vi "while.vi"() -> ()   [LabVIEW 2020]
panel:
  out "Array":dbl[](array[numeric])
  out "Thermometer":dbl(slide) scale=0.0..100.0
  out "Numeric":i32
  in  "stop":bool
  # "While"
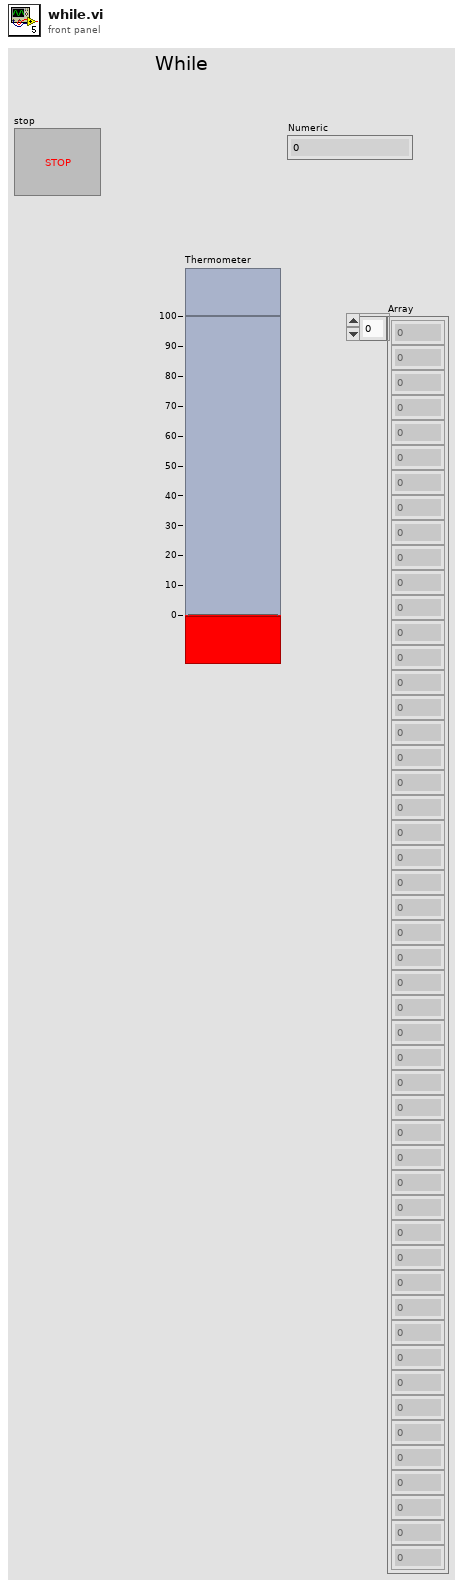
[diagram p1: front panel]
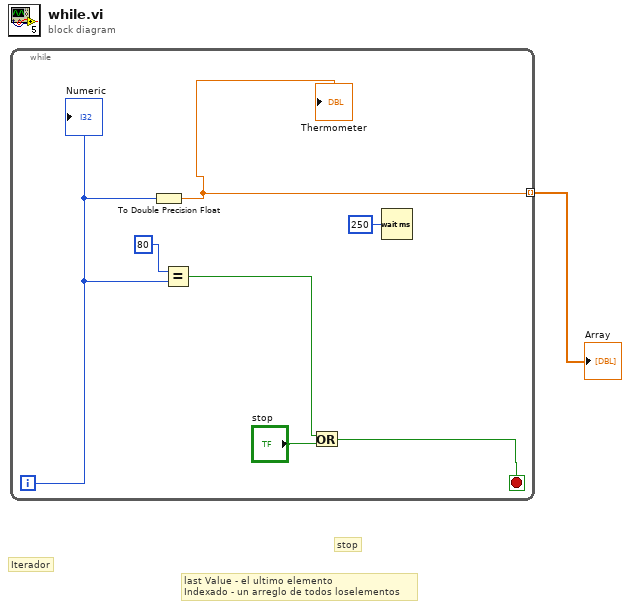
[diagram p0: block diagram]
diagram:
  # "last Value - el ultimo elemento\nIndexado - un arreglo de todos loselementos"
  # "stop"
  # "Iterador"
  n1 = while {
    tunnel: [w2] -> w1 mode=indexing
    i -> [w6]
    stop <- w3 stop-if-true
    n2 = To Double Precision Float(number=w6) -> (double precision float=w2:dbl)
    "Thermometer" <- w2
    n3 = Equal?(x=80, y=w6) -> (x = y?=w4:bool)
    n4 = Or(x=w4, y="stop") -> (x .or. y?=w3:bool)
    n5 = Wait (ms)(milliseconds to wait=u32 250) -> ()  [unwired: 1 out]
    "Numeric" <- w6
  }
  "Array" <- w1
